vi "DSF.Engine.Framework.Initialize.Plugins.vi"(8 "error in (no error)":errorcluster, 11 "Framework in":refnum<class "DSF.Engine.Framework.lvclass">) -> (0 "error out":errorcluster, 3 "Framework out":refnum<class "DSF.Engine.Framework.lvclass">)   [LabVIEW 2017, in "DSF.Engine.lvlib" / "DSF.Engine.Framework.lvclass"]
uses:
  DSF.Engine.Framework.lvclass
  Plugin/DSF.Engine.Plugin.lvclass
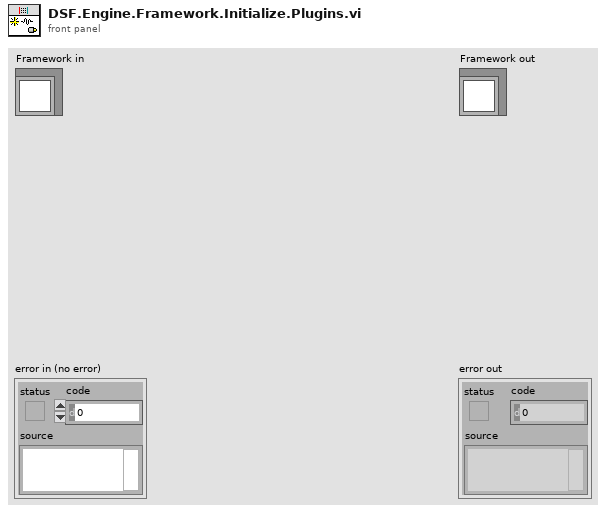
[diagram p1: front panel]
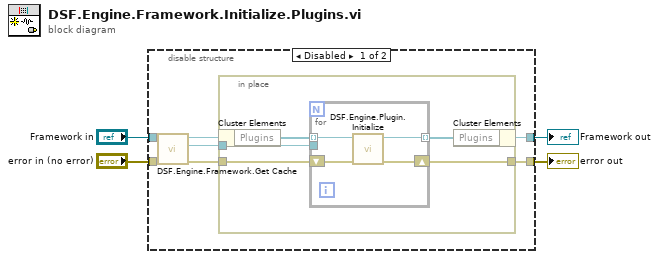
[diagram p0: block diagram]
diagram:
  n1 = disable-structure shown="Disabled" {
    disable-tunnel: [w10 w20] -> w4
    disable-tunnel: "error in (no error)" -> [w9 w20]
    disable-tunnel: [w6 w21] -> w2
    disable-tunnel: "Framework in" -> [w5 w21]
    frame Disabled {
      n2 = call "DSF.Engine.Framework.Get Cache.vi"("Framework in"=w5) -> ("Cache"=w8:refnum<class "DSF.Engine.Memory.Cache.lvclass">, "Framework out"=w7:refnum<class "DSF.Engine.Framework.lvclass">)  [unwired: 9 in]
      n3 = in-place {
        in-place-border: [w15] -> w10
        in-place-border: w9 -> [w14]
        in-place-border: w8 -> [w13]
        n4 = in-place-cluster #1(w7) -> ("Plugins"=w12:refnum<class "DSF.Engine.Plugin.lvclass">[])
        n5 = for {
          tunnel: w12 -> [w19] mode=indexing
          tunnel: [w18] -> w11 mode=indexing
          shift-right: [w17] -> w15
          shift-left: w14 -> [w16]
          tunnel: w13 -> [_]
          n6 = call "DSF.Engine.Plugin.Initialize.vi"("error in (no error)"=w16, "Plugin in"=w19) -> ("error out"=w17:errorcluster, "Plugin out"=w18:refnum<class "DSF.Engine.Plugin.lvclass">)  [unwired: 8 in]
        }
        n7 = in-place-cluster #1("Plugins"=w11) -> (w6:refnum<class "DSF.Engine.Framework.lvclass">)
      }
    }
    frame Enabled {
    }
  }
  "error out" <- w4
  "Framework out" <- w2
